vi "Communications test.vi"() -> ()   [LabVIEW 2022 SP3]
panel:
  out "2":bool=TRUE
  out "1":bool=TRUE
  in  "stop":bool
  out "Robot message":string
  out "error Read 2":errorcluster
  in  "Write or listen":bool
  out "error Read":errorcluster
  out "error Second send, order":errorcluster
  out "error First send, string lengh":errorcluster
  in  "Order":string="(0,0,0,0,0,0,0,0,0)"
  out "error out":errorcluster
  out "connection ID out":refnum<k5>
  in  "port":u16=30002
  in  "service name":string="192.168.0.10"
  # "Write to the robot"
  # "Listen to the robot"
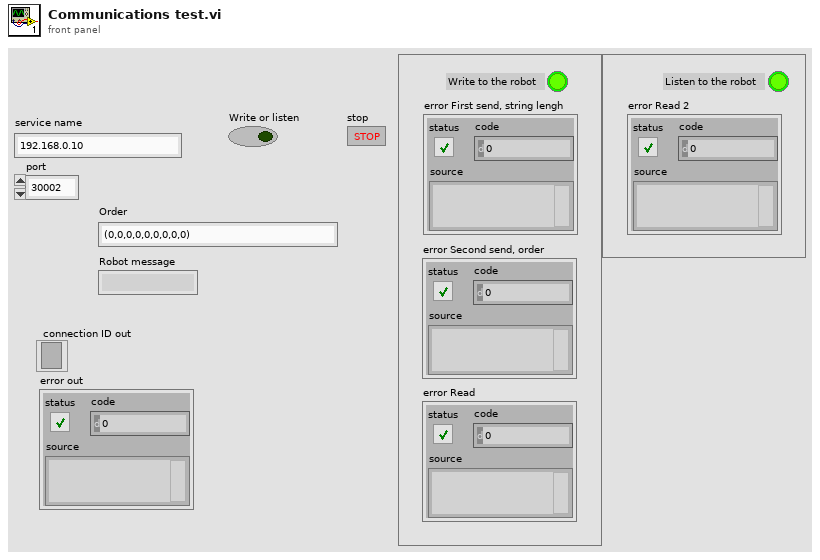
[diagram p1: front panel]
types:
  T1 = enum16{"Standard", "Buffered", "CRLF", "Immediate"}
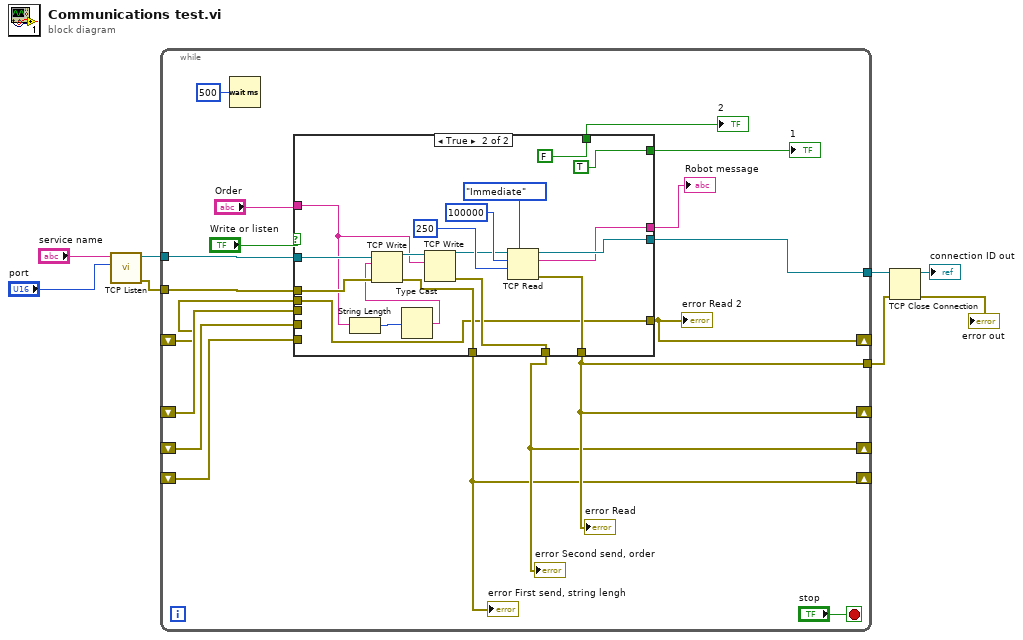
[diagram p0: block diagram]
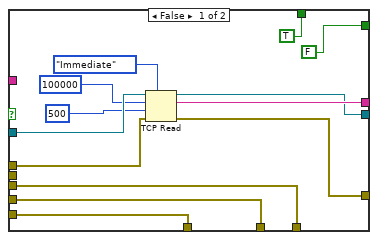
[diagram p2: hidden frame]
diagram:
  n1 = call <vilib>:"TCP Listen.vi"("port"="port", "service name"="service name") -> ("error out"=w8:errorcluster, "connection ID"=w7:refnum<k5>)  [unwired: 5 in, 3 out]
  n2 = while {
    tunnel: w8 -> [w26]
    tunnel: w7 -> [w25]
    tunnel: [w24] -> w2
    tunnel: [w21] -> w1
    shift-right: [w21] -> _
    shift-left: _ -> [w18]
    shift-right: [w20] -> _
    shift-left: _ -> [w17]
    shift-right: [w19] -> _
    shift-left: _ -> [w16]
    shift-right: [w14] -> _
    shift-left: _ -> [w13]
    stop <- "stop" stop-if-true
    n3 = Wait (ms)(milliseconds to wait=u32 500) -> ()  [unwired: 1 out]
    n4 = case shown="True" "Write or listen" {
      tunnel: w26 -> [w38 w52]
      tunnel: w25 -> [w39 w51]
      tunnel: [w27 w50] -> w24
      tunnel: "Order" -> [_ w49]
      tunnel: [w35 w46] -> w19
      tunnel: [w36 w45] -> w20
      tunnel: [w37 w44] -> w21
      tunnel: w18 -> [w37 _]
      tunnel: w17 -> [w36 _]
      tunnel: w16 -> [w35 _]
      tunnel: [w34 w43] -> w14
      tunnel: [w33 w40] -> w15
      tunnel: w13 -> [_ w43]
      tunnel: [TRUE FALSE] -> w10
      tunnel: [FALSE TRUE] -> w9
      frame False {
        n5 = TCP Read(connection ID=w39, bytes to read=100000, error in (no error)=w38, 7:T1."Immediate" ("mode (standard)"), 9:500 ("timeout ms (25000)")) -> (connection ID out=w27:refnum<k5>, data out=w33:string, error out=w34:errorcluster)
      }
      frame True {
        n6 = String Length(string=w49) -> (length=w48:i32)
        n7 = Type Cast(x=w48) -> (*(type *) &x=w47:string)  [unwired: 1 in]
        n8 = TCP Write(connection ID=w51, data in=w47, error in (no error)=w52) -> (connection ID out=w53:refnum<k5>, error out=w46:errorcluster)  [unwired: 1 in, 1 out]
        n9 = TCP Write(connection ID=w53, data in=w49) -> (connection ID out=w54:refnum<k5>, error out=w45:errorcluster)  [unwired: 2 in, 1 out]
        n10 = TCP Read(connection ID=w54, bytes to read=100000, 7:T1."Immediate" ("mode (standard)"), 9:250 ("timeout ms (25000)")) -> (connection ID out=w50:refnum<k5>, data out=w40:string, error out=w44:errorcluster)  [unwired: 1 in]
      }
    }
    "error First send, string lengh" <- w19
    "error Second send, order" <- w20
    "error Read" <- w21
    "error Read 2" <- w14
    "Robot message" <- w15
    "2" <- w10
    "1" <- w9
  }
  n11 = TCP Close Connection(connection ID=w2, error in (no error)=w1) -> (connection ID out=→"connection ID out":refnum<k5>, error out=→"error out":errorcluster)  [unwired: 1 in]
